vi "Volatus Pre-Build Action.vi"(6 "Top Level/Always Included VIs":path[](array[path]), 7 "Main Destination Path":path, 9 "Target Name":string, 10 "Build Specification Name":string, 11 "Project Path":path) -> (0 "error out":errorcluster)   [LabVIEW 2020, in "VolatusBuild.lvlib"]
uses:
  VolatusBuild.lvlib
  <vilib>/AppBuilder/AB_API_Simple/Get Build Specification Version (path).vi
  <vilib>/AppBuilder/AB_API_Simple/NI_App_Builder_API.lvlib
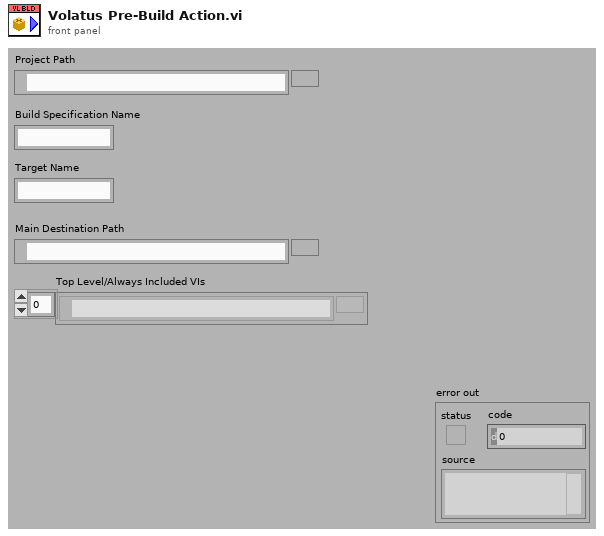
[diagram p1: front panel]
types:
  T1 = typedef "NI_App_Builder_API.lvlib/Build Specification Version.ctl" = cluster{"Major":u16, "Minor":u16, "Fix":u16, "Build":u16}
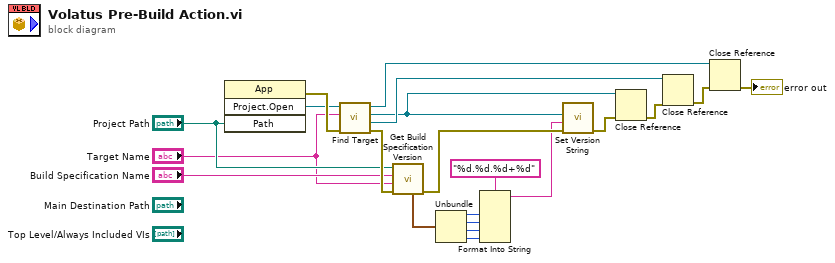
[diagram p0: block diagram]
diagram:
  n1 = invoke class="App" method="Project.Open"("Path"="Project Path") -> (error out=w20:errorcluster, "Project:Open"=w19:refnum<vi>)  [unwired: 3 in, 2 out]
  n2 = call "Find Target.vi"("error in (no error)"=w20, "Target"="Target Name", "Project in"=w19) -> ("error out"=w21:errorcluster, "Target"=w8:refnum<vi>, "TargetAppContext"=w3:refnum<vi>, "Project"=w6:refnum<vi>)  [unwired: 5 in]
  n3 = call-poly <vilib>:"Get Build Specification Version.vi"("error in (no error)"=w21, "Name of target (My Computer)"="Target Name", "Name of build specification"="Build Specification Name", "Path to project"="Project Path") -> ("error out"=w4:errorcluster, "Build Specification Version"=w15:T1)  [unwired: 6 in]
  n4 = Unbundle(w15) -> ("Major"=w13:u16, "Minor"=w12:u16, "Fix"=w11:u16, "Build"=w10:u16)
  n5 = Format Into String(format string="%d.%d.%d+%d", w13, w12, w11, w10) -> (resulting string=w2:string)  [unwired: 2 in, 1 out]
  n6 = call "Set Version String.vi"("error in (no error)"=w4, "Version String"=w2, "App"=w3) -> ("error out"=w1:errorcluster)  [unwired: 8 in]
  n7 = Close Reference(reference=w3, error in (no error)=w1) -> (error out=w9:errorcluster)
  n8 = Close Reference(reference=w8, error in (no error)=w9) -> (error out=w7:errorcluster)
  n9 = Close Reference(reference=w6, error in (no error)=w7) -> (error out=→"error out":errorcluster)
